vi "FGV Schedule Status.vi"(11 "error in (no error)":errorcluster caption="Fehler (Eingang, kein Fehler)", 13 "Aktion":T1) -> (4 "Scheduler Status":bool, 15 "error out":errorcluster caption="Fehler (Ausgang)")   [LabVIEW 2020, in "Schedule Modul.lvlib"]
uses:
  Schedule Modul.lvlib
  Aktion FGV Scheduler Status.ctl
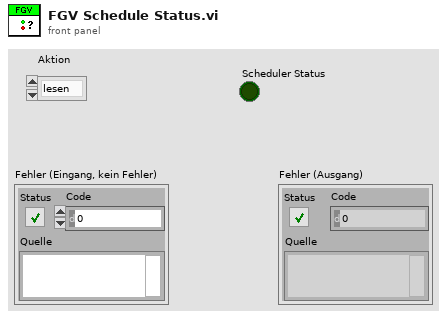
[diagram p1: front panel]
types:
  T1 = typedef "Schedule Modul.lvlib/Aktion FGV Scheduler Status.ctl" = enum16{"lesen", "init", "aktiv", "inaktiv"}
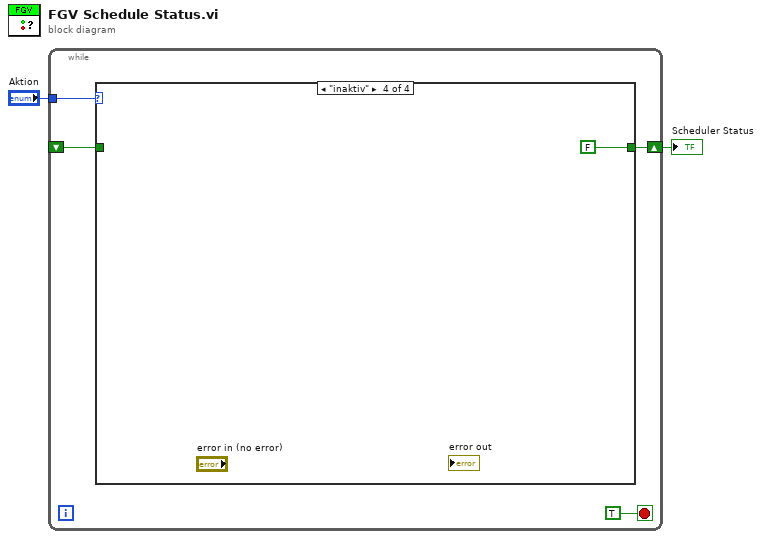
[diagram p0: block diagram]
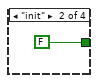
[diagram p3: hidden frame]
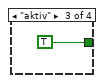
[diagram p4: hidden frame]
diagram:
  n1 = while {
    tunnel: "Aktion" -> [w5]
    shift-right: [w4] -> w2
    shift-left: _ -> [w3]
    stop <- TRUE stop-if-true
    n2 = case shown="\"inaktiv\"" w5 {
      tunnel: [w7 FALSE TRUE FALSE] -> w4
      tunnel: w3 -> [w7 _ _ _]
      frame "lesen", Default {
      }
      frame "init" {
      }
      frame "aktiv" {
      }
      frame "inaktiv" {
      }
    }
  }
  "Scheduler Status" <- w2
